vi "example.vi"() -> ()   [LabVIEW 2017]
uses:
  models/DPF_operationMode.ctl
  tools/subvi/DPF.vi
  tools/subvi/dpfOperationModeData.vi
panel:
  out "error out":errorcluster caption="errorOut"
  in  "errorIn":errorcluster
  out "OperationMode":T1
  out "shotNum":string
  in  "nodeName":string
  in  "xmlFilePath":path
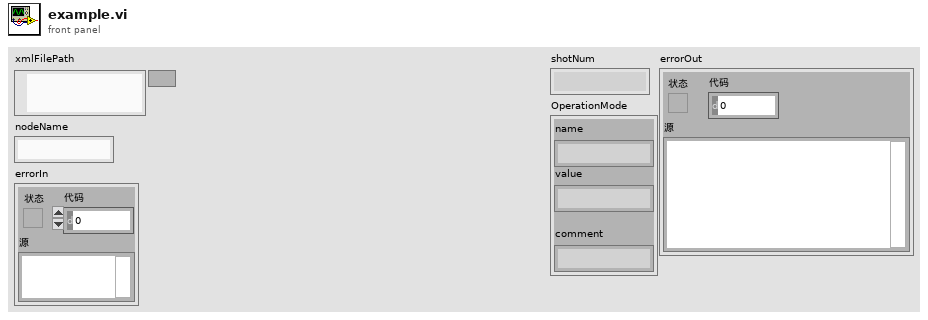
[diagram p1: front panel]
types:
  T1 = typedef "DPF_operationMode.ctl" = cluster{"name":string, "value":string, "comment":string}
  T2 = typedef "DPF.ctl" = cluster{"Header":T3, "ocpeo":T4}
  T3 = typedef "Header.ctl" = cluster{"version":string, "operator":string, "shotnum":string}
  T4 = typedef "DPF_ocpeo.ctl" = cluster{"OperationModes":T1[], "Commands":T5[], "PIDcontrollers":T6[], "EngineLimits":T7[], "Others":T8[]}
  T5 = typedef "DPF_command.ctl" = cluster{"name":string, "value":string, "personInCharge":string, "implementationHistory":string, "db":string, "comment":string}
  T6 = typedef "DPF_pidController.ctl" = cluster{"Name":string, "P":string, "I":string, "D":string, "RC":string, "MaxdU":string, "FBStart":string, "maxInvAngle":string, "personInCharge":string, "implementationHistory":string, "comment":string}
  T7 = typedef "DPF_engineLimit.ctl" = cluster{"Name":string, "Value":string, "personInCharge":string, "implementationHistory":string, "comment":string}
  T8 = typedef "DPF_other.ctl" = cluster{"name":string, "value":string, "remark":string}
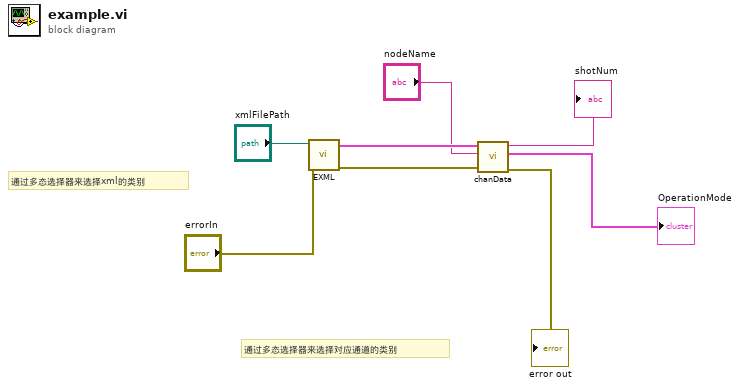
[diagram p0: block diagram]
diagram:
  # "通过多态选择器来选择对应通道的类别"
  # "通过多态选择器来选择xml的类别"
  n1 = call-poly "EXML.vi"("errorIn"="errorIn", "xmlFilePath"="xmlFilePath") -> ("error out"=w3:errorcluster, "DPF"=w7:T2)  [unwired: 8 in]
  n2 = call-poly "chanData.vi"("errorIn"=w3, "nodeName"="nodeName", "DPF"=w7) -> ("error out"=→"error out":errorcluster, "OperationMode"=→"OperationMode":T1, "shotNum"=→"shotNum":string)  [unwired: 6 in]
